vi "S2C_LogProcError.vi"(8 "Error In":errorcluster, 10 "Error Details":string[](array[string]), 11 "Error Msg":string) -> (0 "Error Out":errorcluster)   [LabVIEW 2024]
doc: "Writes the error text to an error file, not to exceed 500 records. Once the limit is reached, the oldest entries will be overwritten first."
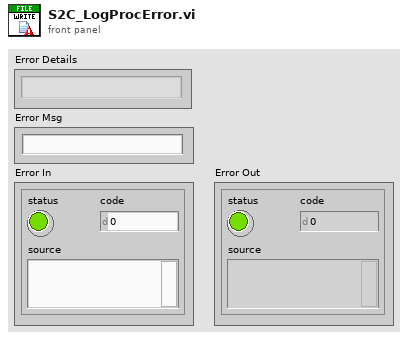
[diagram p1: front panel]
types:
  T1 = enum16{"open", "replace", "create", "open or create", "replace or create", "replace or create with confirmation"}
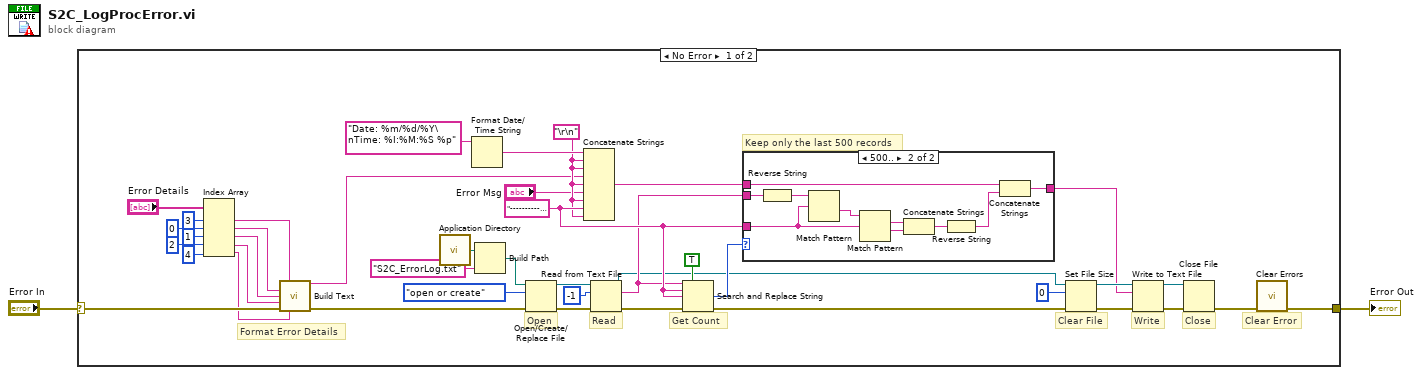
[diagram p0: block diagram]
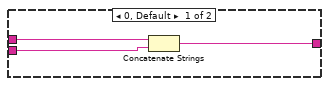
[diagram p2: hidden frame]
diagram:
  n1 = case shown="No Error" "Error In" {
    selector: "Error In" -> [w18 w57]
    tunnel: [w26 w57] -> w2
    frame No Error {
      w40 = "----------------------------------------------------------------------------------------------------"
      w16 = "\r\n"
      # "Format Error Details"
      # "Clear Error"
      # "Get Count"
      # "Keep only the last 500 records"
      # "Write"
      # "Clear File"
      # "Close"
      # "Read"
      # "Open"
      n2 = Index Array(array="Error Details", index #1=3 ("index"), index #2=0 ("index"), index #3=1 ("index"), index #4=2 ("index"), index #5=4 ("index")) -> (element #1=w14:string, element #2=w11:string, element #3=w9:string, element #4=w8:string, element #5=w6:string)
      n3 = call "Build Text"("Call"=w14, "Process"=w11, "Cmd"=w9, "Driver"=w8, "error in (no error)"=w18, "Code"=w6) -> ("Result"=w15:string, "error out"=w17:errorcluster)  [unwired: 8 in]
      n4 = call <vilib>:"Application Directory.vi"() -> ("Application Directory"=w21:path)
      n5 = Format Date/Time String(time format string (%c)="Date: %m/%d/%Y\nTime: %I:%M:%S %p") -> (date/time string=w28:string)  [unwired: 2 in]
      n6 = Build Path(base path=w21, name or relative path="S2C_ErrorLog.txt") -> (appended path=w19:path)
      n7 = Open/Create/Replace File(file path (use dialog)=w19, error in=w17, operation (0:open)=T1."open or create") -> (refnum out=w31:refnum<file>, error out=w32:errorcluster)  [unwired: 3 in, 1 out]
      n8 = Concatenate Strings(w28, w16, w16, w15, w16, "Error Msg", w16, w40, w16) -> (w24:string)
      n9 = Read from Text File(file (use dialog)=w31, count=-1, error in=w32) -> (refnum out=w23:refnum<file>, text=w39:string, error out=w38:errorcluster)  [unwired: 1 in, 1 out]
      n10 = Search and Replace String(replace all?=TRUE ("replace all? (F)"), input string=w39, search string=w40, replace string=w40, error in=w38) -> (number of replacements=w43:i32, error out=w42:errorcluster)  [unwired: 3 in, 2 out]
      n11 = case shown="500.." w43 {
        tunnel: [w44 w53] -> w25
        tunnel: w39 -> [w45 w56]
        tunnel: w40 -> [_ w50]
        tunnel: w24 -> [w46 w54]
        frame 0, Default {
          n12 = Concatenate Strings(w46, w45) -> (w44:string)
        }
        frame 500.. {
          n13 = Reverse String(1:w56) -> (0:w52:string)
          n14 = Match Pattern(string=w52, regular expression=w50) -> (after substring=w51:string)  [unwired: 1 in, 3 out]
          n15 = Match Pattern(string=w51, regular expression=w50) -> (match substring=w48:string, after substring=w49:string)  [unwired: 1 in, 2 out]
          n16 = Concatenate Strings(w48, w49) -> (w47:string)
          n17 = Reverse String(1:w47) -> (0:w55:string)
          n18 = Concatenate Strings(w54, w55) -> (w53:string)
        }
      }
      n19 = Set File Size(4:w42, 6:i64 0 ("offset (in bytes) (0)"), 7:w23) -> (0:w34:errorcluster, 3:w35:refnum<file>)
      n20 = Write to Text File(file (use dialog)=w35, text=w25, error in=w34) -> (refnum out=w37:refnum<file>, error out=w36:errorcluster)  [unwired: 1 in, 1 out]
      n21 = Close File(refnum=w37, error in=w36) -> (error out=w27:errorcluster)  [unwired: 1 out]
      n22 = call <vilib>:"Clear Errors.vi"("error in (no error)"=w27) -> ("error out"=w26:errorcluster)  [unwired: 5 in, 1 out]
    }
    frame Error {
    }
  }
  "Error Out" <- w2
